vi "open connection.vi"(6 "timeout ms (10000)":i32=10000, 8 "error in":errorcluster, 10 "process ID":string, 11 "address":string) -> (0 "error out":errorcluster, 2 "valid?":bool, 3 "output cluster":T1)   [LabVIEW 2015, in "Queue client.lvclass"]
uses:
  Queue client.lvclass
  Queue connection/queue pair.ctl
  message/communicator message.lvclass
  opening handshake data.ctl
  message/communicator message.lvclass/communicator message.ctl
  Queue connection/Queue connection.lvclass
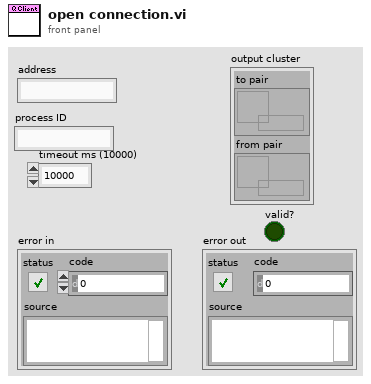
[diagram p1: front panel]
types:
  T1 = typedef "Queue connection.lvclass/queue pair.ctl" = cluster{"to pair":refnum<queue>, "from pair":refnum<queue>}
  T2 = typedef "Queue client.lvclass/opening handshake data.ctl" = cluster{"queue":refnum<queue>, "process ID":string}
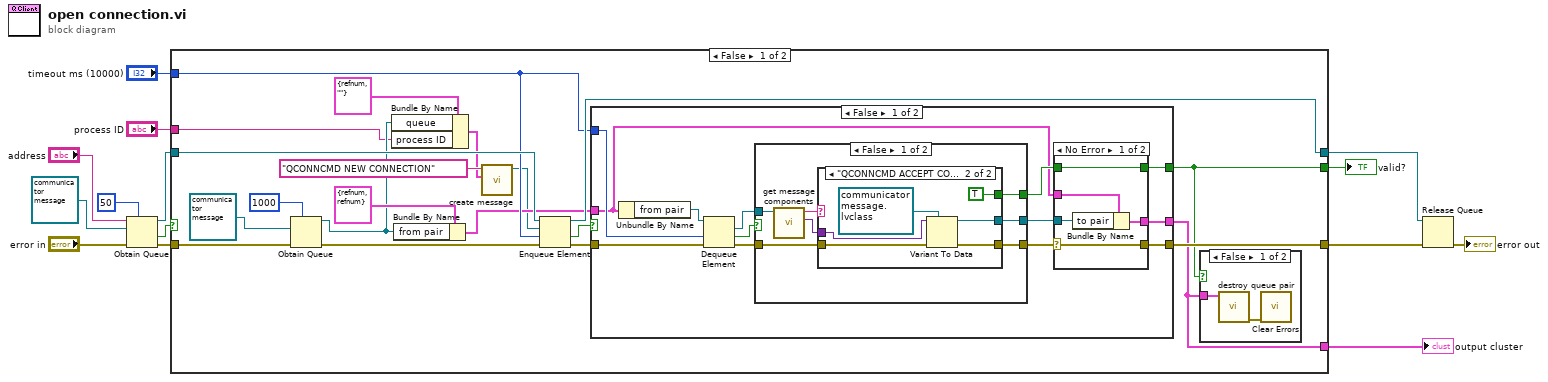
[diagram p0: block diagram]
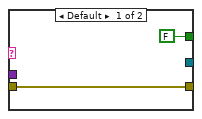
[diagram p4: hidden frame]
diagram:
  n1 = Obtain Queue(max queue size (-1, unlimited)=50, name (unnamed)="address", element data type=refnum<class "communicator message.lvclass"> refnum ("communicator message.lvclass"), error in (no error)="error in") -> (queue out=w10:refnum<queue>, created new?=w5:bool, error out=w11:errorcluster)  [unwired: 1 in]
  n2 = case shown="False" w5 {
    tunnel: w11 -> [w28 w73]
    tunnel: w10 -> [w34 w74]
    tunnel: [w31 w73] -> w9
    tunnel: [w30 w74] -> w7
    tunnel: [w23 _] -> w4
    tunnel: [w22 _] -> w3
    tunnel: "timeout ms (10000)" -> [w29 _]
    tunnel: "process ID" -> [w15 _]
    frame False {
      n3 = Obtain Queue(max queue size (-1, unlimited)=1000, element data type=refnum<class "communicator message.lvclass"> refnum ("communicator message.lvclass"), error in (no error)=w28) -> (queue out=w17:refnum<queue>, error out=w27:errorcluster)  [unwired: 2 in, 1 out]
      n4 = Bundle By Name(cluster=T2 {"queue"=refnum, "process ID"=""} ("handshake data"), "queue"=w17, "process ID"=w15) -> (w16:T2)
      n5 = Bundle By Name(cluster=T1 {"to pair"=refnum, "from pair"=refnum} ("queues"), "from pair"=w17) -> (w24:T1)
      n6 = call "create message.vi"("data"=w16, "ID"="QCONNCMD NEW CONNECTION") -> ("message"=w19:refnum<class "communicator message.lvclass">)  [unwired: 9 in]
      n7 = Enqueue Element(queue=w34, element=w19, timeout in ms (-1)=w29, error in (no error)=w27) -> (queue out=w30:refnum<queue>, timed out?=w32:bool, error out=w33:errorcluster)
      n8 = case shown="False" w32 {
        tunnel: w33 -> [w49 w72]
        tunnel: [w41 w72] -> w31
        tunnel: w29 -> [w46 _]
        tunnel: [w43 _] -> w23
        tunnel: [w40 _] -> w22
        tunnel: w24 -> [w38 _]
        frame False {
          n9 = Unbundle By Name(w38) -> ("from pair"=w37:refnum<queue>)
          n10 = Dequeue Element(queue=w37, timeout in ms (-1)=w46, error in (no error)=w49) -> (element=w47:refnum<class "communicator message.lvclass">, timed out?=w45:bool, error out=w48:errorcluster)  [unwired: 1 out]
          n11 = case shown="False" w45 {
            tunnel: w48 -> [w62 w71]
            tunnel: w47 -> [w58 _]
            tunnel: [w61 w71] -> w44
            tunnel: [w60 _] -> w42
            tunnel: [w59 _] -> w39
            frame False {
              n12 = call "get message components.vi"("message"=w58) -> ("data"=w57:variant, "ID"=w56:string)  [unwired: 9 in]
              n13 = case shown="\"QCONNCMD ACCEPT CONNECTION\"" w56 {
                tunnel: w62 -> [w63 w70]
                tunnel: [w63 w69] -> w61
                tunnel: [_ w68] -> w60
                tunnel: [FALSE TRUE] -> w59
                tunnel: w57 -> [_ w65]
                frame Default {
                }
                frame "QCONNCMD ACCEPT CONNECTION" {
                  n14 = Variant To Data(error in=w70, type=refnum<queue> refnum ("to pair"), Variant=w65) -> (data=w68:refnum<queue>, error out=w69:errorcluster)
                }
              }
            }
            frame True {
            }
          }
          n15 = case shown="No Error" w44 {
            selector: w44 -> [w54 w55]
            tunnel: [w50 _] -> w43
            tunnel: w42 -> [w51 _]
            tunnel: [w54 w55] -> w41
            tunnel: [w53 _] -> w40
            tunnel: w39 -> [w53 _]
            tunnel: w38 -> [w52 _]
            frame No Error {
              n16 = Bundle By Name(cluster=w52, "to pair"=w51) -> (w50:T1)
            }
            frame Error {
            }
          }
        }
        frame True {
        }
      }
      n17 = case shown="False" w22 {
        tunnel: w23 -> [w36 _]
        frame False {
          n18 = call "destroy queue pair.vi"("queue connection"=w36) -> ("error out"=w35:errorcluster)  [unwired: 10 in]
          n19 = call <vilib>:"Clear Errors.vi"("error in (no error)"=w35) -> ()  [unwired: 5 in, 2 out]
        }
        frame True {
        }
      }
    }
    frame True {
    }
  }
  "output cluster" <- w4
  "valid?" <- w3
  n20 = Release Queue(queue=w7, error in (no error)=w9) -> (error out=→"error out":errorcluster)  [unwired: 1 in, 2 out]
